vi "Autonomous Independent.vi"() -> ()   [LabVIEW 2013]
doc: "This VI is called when autonomous begins, and will automatically be terminated when autonomous ends. You can carry out timed or sensor driven robot movement independently without needing to return to the caller."
uses:
  <vilib>/Rock Robotics/WPI/Solenoid/WPI_SolenoidValue.ctl
  Robot Global Data.vi
  Systems/Sensors/Sensors Global Values.vi
  <vilib>/Rock Robotics/WPI/RobotDrive/WPI_RobotDriveArcadeDrive_Standard(NoSaturation).vi
  <vilib>/Rock Robotics/WPI/Solenoid/WPI_SolenoidSetEnum.vi
panel:
  in  "drive forward to collect ball time":u32
  in  "Distance wanted (ft)":dbl=6.0 format="%#_13g"
  in  "Voltage per meter":dbl=0.96992
  # "Be sure to right-click and choose Data Operations>>Make Current Value default if you want to save the array values with the VI"
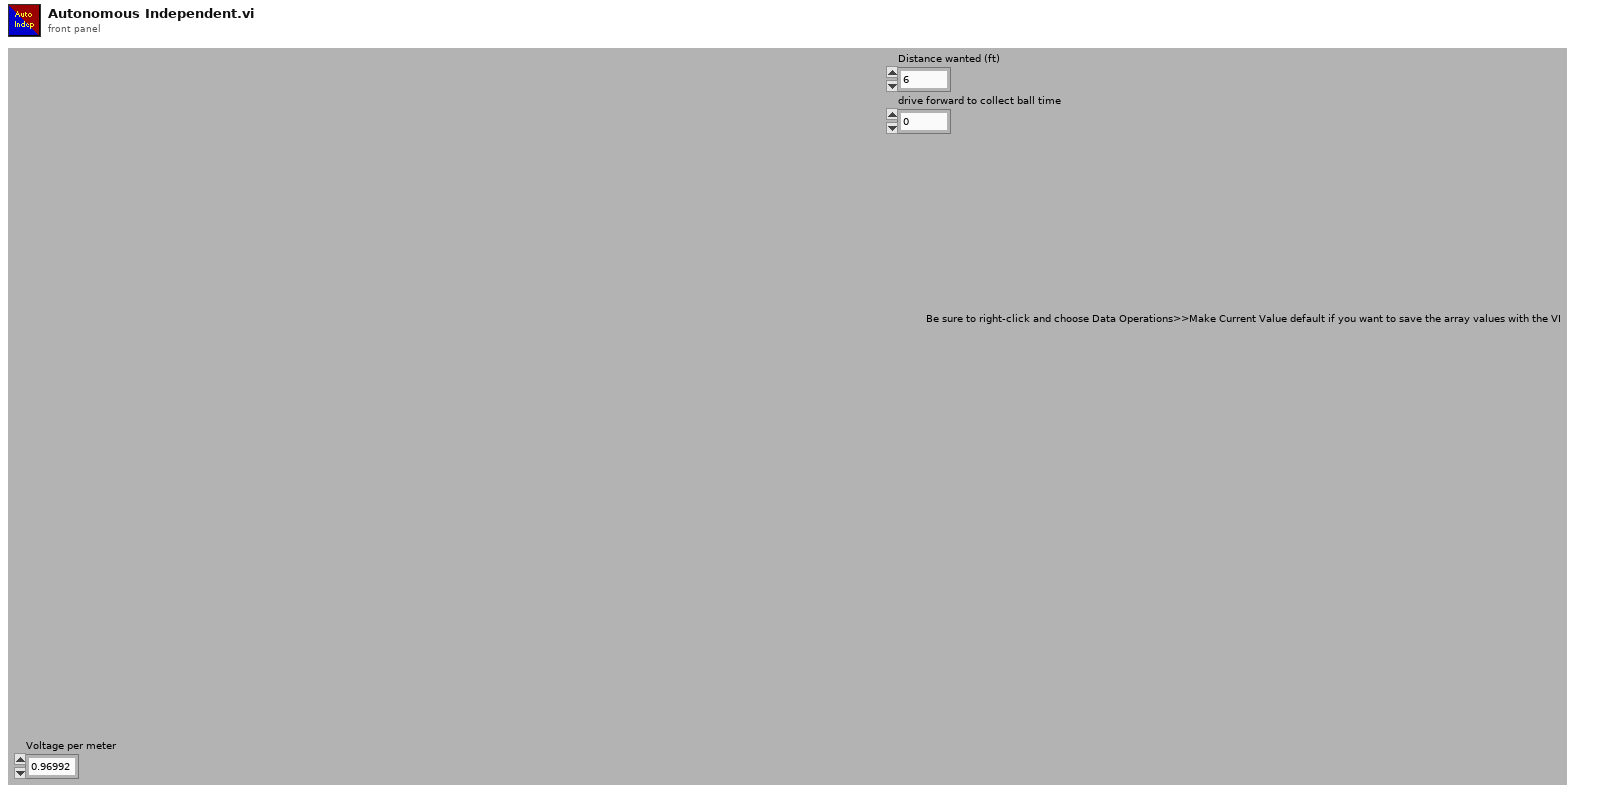
[diagram p1: front panel]
types:
  T1 = typedef "WPI_SolenoidValue.ctl" = enum16{"Off", "On", "Forward", "Reverse"}
  T2 = typedef "WPI_AnalogChannelDevRef.ctl" = cluster{"DevStatus":errorcluster, "Analog Module":T3, "Analog Channel":T4}
  T3 = typedef "FPGA_TypedefAnalogModule.ctl" = enum16{"Analog Module 1", "Analog Module 2"}
  T4 = typedef "FPGA_AIChannel.ctl" = enum8{"AI 1", "AI 2", "AI 3", "AI 4", "AI 5", "AI 6", "AI 7", "AI 8", "Invalid"}
  T5 = typedef "WPI_MotorControlDeviceRef.ctl" = cluster{"DeviceStatus":errorcluster, "Type":enum16{"PWM", "CAN"}, "PWM":cluster{"Digital Module":T6, "PWM Channel":T7, "DeadBand":T8}, "CAN":cluster{"Device Number":u8, "Control Mode":T9, "Semaphore":T10, "Max Vout":dbl}, "Invert":bool, "TransformRef":T11, "InvTransformRef":T11}
  T6 = typedef "FPGA_TypedefDigitalModule.ctl" = enum16{"Digital Module 1", "Digital Module 2"}
  T7 = typedef "FPGA_DIOPWMChannel.ctl" = enum8{"PWM 1", "PWM 2", "PWM 3", "PWM 4", "PWM 5", "PWM 6", "PWM 7", "PWM 8", "PWM 9", "PWM 10", "Invalid"}
  T8 = typedef "WPI_PWMDeadband.ctl" = cluster{"Name":string, "maxPositivePwm":i32, "minPositivePwm":i32, "centerPwm":i32, "maxNegativePwm":i32, "minNegativePwm":i32, "angularRange":u16}
  T9 = typedef "WPI_CANJaguar_ControlMode.ctl" = enum8{"Percent VBus", "Current", "Speed", "Position", "Voltage"}
  T10 = typedef "Semaphore RefNum" = refnum<k1>
  T11 = typedef "WPI_PWMTransform_ConPane.ctl" = refnum<vi>
  T12 = typedef "WPI_DigitalInputDevRef.ctl" = cluster{"DevStatus":errorcluster, "DIO Channel":T13, "Digital Module":T6}
  T13 = typedef "FPGA_DIOChannel.ctl" = enum8{"DIO 1", "DIO 2", "DIO 3", "DIO 4", "DIO 5", "DIO 6", "DIO 7", "DIO 8", "DIO 9", "DIO 10", "DIO 11", "DIO 12", "DIO 13", "DIO 14", "Invalid"}
  T14 = typedef "WPI_RobotDriveDevRef.ctl" = cluster{"DevStatus":errorcluster, "Motors[]":T5[], "Square Inputs":bool, "Max Output":dbl, "Isochronous":bool}
  T15 = typedef "WPI_ServoDeviceRef.ctl" = cluster{"DeviceStatus":errorcluster, "Digital Module":T6, "PWM Channel":T7, "DeadBand":T8}
  T16 = typedef "WPI_SolenoidDevRef.ctl" = cluster{"DevStatus":errorcluster, "Solenoid Module":T17, "Forward Solenoid Channel":T18, "Reverse Solenoid Channel":T18}
  T17 = typedef "FPGA_TypedefSolenoidModule.ctl" = enum16{"Solenoid Module 1", "Solenoid Module 2"}
  T18 = typedef "WPI_SolenoidChannel.ctl" = enum8{"Solenoid 1", "Solenoid 2", "Solenoid 3", "Solenoid 4", "Solenoid 5", "Solenoid 6", "Solenoid 7", "Solenoid 8", "Invalid"}
  T19 = cluster{"Camera Sonar":dbl, "Front Right Sonar":dbl, "Front Left Sonar":dbl, "Rear Sonar":dbl}
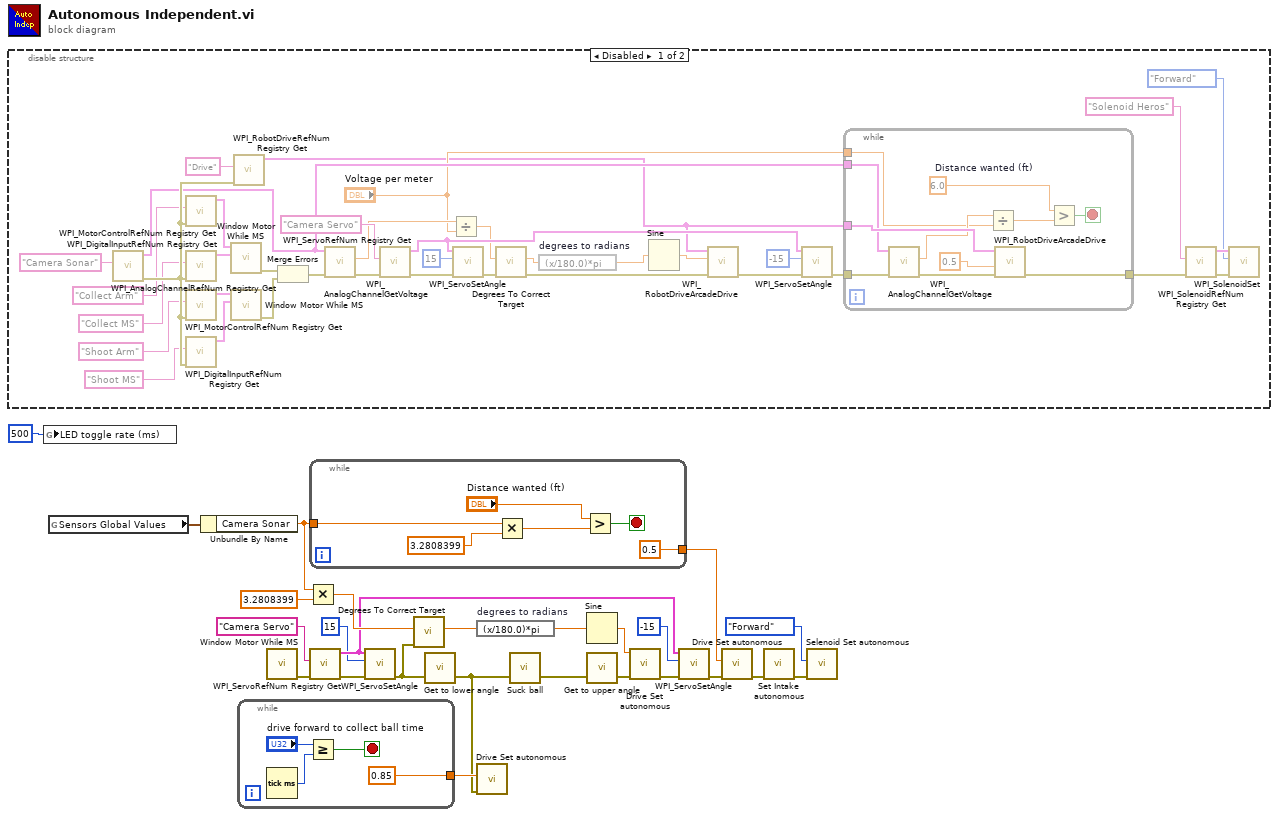
[diagram p0: block diagram]
diagram:
  n1 = disable-structure shown="Disabled" {
    frame Disabled {
      n2 = call <vilib>:"WPI_AnalogChannelRefNum Registry Get.vi"("refnum name"="Camera Sonar") -> ("error out"=w42:errorcluster, "AIDeviceRef"=w37:T2)  [unwired: 9 in]
      n3 = call <vilib>:"WPI_MotorControlRefNum Registry Get.vi"("error in (no error)"=w42, "refnum name"="Collect Arm") -> ("MotorControlDevRef"=w41:T5)  [unwired: 8 in, 1 out]
      n4 = call <vilib>:"WPI_DigitalInputRefNum Registry Get.vi"("error in (no error)"=w42, "refnum name"="Collect MS") -> ("DigitalInputDevRef"=w40:T12)  [unwired: 8 in, 1 out]
      n5 = call <vilib>:"WPI_MotorControlRefNum Registry Get.vi"("error in (no error)"=w42, "refnum name"="Shoot Arm") -> ("MotorControlDevRef"=w39:T5)  [unwired: 8 in, 1 out]
      n6 = call <vilib>:"WPI_DigitalInputRefNum Registry Get.vi"("error in (no error)"=w42, "refnum name"="Shoot MS") -> ("DigitalInputDevRef"=w38:T12)  [unwired: 8 in, 1 out]
      n7 = call "Window Motor While MS.vi"(10:w40, 11:w41) -> ("error out"=w34:errorcluster)  [unwired: 9 in]
      n8 = call "Window Motor While MS.vi"(10:w38, 11:w39) -> ("error out"=w35:errorcluster)  [unwired: 9 in]
      n9 = call <vilib>:"WPI_RobotDriveRefNum Registry Get.vi"("error in (no error)"=w42, "refnum name"="Drive") -> ("RobotDriveDevRef"=w32:T14)  [unwired: 8 in, 1 out]
      n10 = Merge Errors(w34, w35) -> (w33:errorcluster)
      n11 = call <vilib>:"WPI_AnalogChannelGetVoltage.vi"("error in (no error)"=w33, "AIDeviceRef"=w37) -> ("error out"=w47:errorcluster, "Voltage"=w46:dbl)  [unwired: 7 in, 1 out]
      n12 = call <vilib>:"WPI_ServoRefNum Registry Get.vi"("error in (no error)"=w47, "refnum name"="Camera Servo") -> ("error out"=w61:errorcluster, "ServoDeviceRef"=w54:T15)  [unwired: 8 in]
      n13 = Divide(x=w46, y="Voltage per meter") -> (x/y=w45:dbl)
      n14 = call <vilib>:"WPI_ServoSetAngle.vi"("error in (no error)"=w61, "Angle"=15, "ServoDeviceRef"=w54) -> ("error out"=w59:errorcluster)  [unwired: 7 in, 1 out]
      n15 = call "Degrees To Correct Target.vi"("error in"=w59, "Distance to Wall (ft)"=w45) -> ("error out"=w43:errorcluster, "Degrees"=w58:dbl)  [unwired: 8 in]
      n16 = expression code="(x/180.0)*pi" "degrees to radians"(w58) -> (w57:dbl)
      n17 = Sine(x=w57) -> (sin(x)=w49:dbl)
      n18 = call-poly <vilib>:"WPI_RobotDriveArcadeDrive.vi"("error in (no error)"=w43, "X axis value"=w49, "RobotDriveDevRef"=w32) -> ("error out"=w56:errorcluster)  [unwired: 6 in, 2 out]
      n19 = call <vilib>:"WPI_ServoSetAngle.vi"("error in (no error)"=w56, "Angle"=-15, "ServoDeviceRef"=w54) -> ("error out"=w48:errorcluster)  [unwired: 7 in, 1 out]
      n20 = while {
        tunnel: w32 -> [w72]
        tunnel: [w67] -> w51
        tunnel: w48 -> [w70]
        tunnel: w37 -> [w69]
        tunnel: "Voltage per meter" -> [w63]
        stop <- w64 stop-if-true
        w66 = 6.0  # Distance wanted (ft)
        n21 = call <vilib>:"WPI_AnalogChannelGetVoltage.vi"("error in (no error)"=w70, "AIDeviceRef"=w69) -> ("error out"=w71:errorcluster, "Voltage"=w68:dbl)  [unwired: 7 in, 1 out]
        n22 = Divide(x=w68, y=w63) -> (x/y=w65:dbl)
        n23 = call-poly <vilib>:"WPI_RobotDriveArcadeDrive.vi"("error in (no error)"=w71, "Y axis value"=0.5, "RobotDriveDevRef"=w72) -> ("error out"=w67:errorcluster)  [unwired: 6 in, 2 out]
        n24 = Greater?(x=w66, y=w65) -> (0:w64:bool)
      }
      n25 = call <vilib>:"WPI_SolenoidRefNum Registry Get.vi"("error in (no error)"=w51, "refnum name"="Solenoid Heros") -> ("error out"=w52:errorcluster, "SolenoidDevRef"=w53:T16)  [unwired: 8 in]
      n26 = call-poly <vilib>:"WPI_SolenoidSet.vi"("error in (no error)"=w52, "Value"=WPI_SolenoidValue."Forward", "SolenoidDevRef"=w53) -> ()  [unwired: 7 in, 2 out]
    }
    frame Enabled {
    }
  }
  n27 = global write "Robot Global Data.vi" "LED toggle rate (ms)"(u32 500 ("LED ms toggle rate")) -> ()
  n28 = global read "Sensors Global Values.vi" "Sensors Global Values"() -> (w24:T19)
  n29 = Unbundle By Name(w24) -> ("Camera Sonar"=w17:dbl)
  n30 = while {
    tunnel: [0.85 ("Y value")] -> w15
    stop <- w75 stop-if-true
    n31 = Tick Count (ms)() -> (millisecond timer value=w77:u32)
    n32 = Greater Or Equal?(x="drive forward to collect ball time", y=w77) -> (x >= y?=w75:bool)
  }
  n33 = call "Window Motor While MS.vi"() -> ("error out"=w5:errorcluster)  [unwired: 11 in]
  n34 = Multiply(x=w17, y=3.2808399) -> (x*y=w16:dbl)
  n35 = while {
    tunnel: w17 -> [w80]
    tunnel: [0.5 ("Y axis value")] -> w21
    stop <- w82 stop-if-true
    n36 = Multiply(x=w80, y=3.2808399) -> (x*y=w78:dbl)
    n37 = Greater?(x="Distance wanted (ft)", y=w78) -> (0:w82:bool)
  }
  n38 = call <vilib>:"WPI_ServoRefNum Registry Get.vi"("error in (no error)"=w5, "refnum name"="Camera Servo") -> ("error out"=w4:errorcluster, "ServoDeviceRef"=w9:T15)  [unwired: 8 in]
  n39 = call <vilib>:"WPI_ServoSetAngle.vi"("error in (no error)"=w4, "Angle"=15, "ServoDeviceRef"=w9) -> ("error out"=w3:errorcluster)  [unwired: 7 in, 1 out]
  n40 = call "Degrees To Correct Target.vi"("error in"=w3, "Distance to Wall (ft)"=w16) -> ("Degrees"=w22:dbl)  [unwired: 8 in, 1 out]
  n41 = call "Get to lower angle.vi"("error in (no error)"=w3) -> ("error out"=w13:errorcluster)  [unwired: 2 in]
  n42 = expression code="(x/180.0)*pi" "degrees to radians"(w22) -> (w23:dbl)
  n43 = call "Drive Set autonomous.vi"("error in (no error)"=w13, "Y value"=w15) -> ()  [unwired: 9 in, 1 out]
  n44 = call "Suck ball.vi"("error in (no error)"=w13) -> ("error out"=w14:errorcluster)  [unwired: 2 in]
  n45 = Sine(x=w23) -> (sin(x)=w20:dbl)
  n46 = call "Get to upper angle.vi"("error in (no error)"=w14) -> ("error out"=w12:errorcluster)  [unwired: 2 in]
  n47 = call "Drive Set autonomous.vi"("error in (no error)"=w12, "X value"=w20) -> ("error out (no error)"=w2:errorcluster)  [unwired: 9 in]
  n48 = call <vilib>:"WPI_ServoSetAngle.vi"("error in (no error)"=w2, "Angle"=-15, "ServoDeviceRef"=w9) -> ("error out"=w1:errorcluster)  [unwired: 7 in, 1 out]
  n49 = call "Drive Set autonomous.vi"("error in (no error)"=w1, "Y value"=w21) -> ("error out (no error)"=w11:errorcluster)  [unwired: 9 in]
  n50 = call "Set Intake autonomous.vi"("error in (no error)"=w11) -> ("error out"=w10:errorcluster)  [unwired: 10 in]
  n51 = call "Selenoid Set autonomous.vi"("error in (no error)"=w10, "Value"=WPI_SolenoidValue."Forward") -> ()  [unwired: 9 in, 1 out]
